vi "RT Main.vi"() -> ()   [LabVIEW 2021]
doc: "Demonstrates the use of Transmission Control Protocol (TCP) to continuously receive LED status from the host computer."
uses:
  <vilib>/myRIO/Express VI/Onboard Devices/LED/LED Express VI.xnode
  <vilib>/myRIO/Instrument Drivers/Onboard IO/DIO/vis/Write.vi
  <vilib>/myRIO/Instrument Drivers/Onboard IO/DIO/DIO.lvlib
  <vilib>/myRIO/Common/Instrument Driver Framework/myRIO v1.0/DIO/typedefs/DIO Channels Enum.ctl
  <vilib>/myRIO/Common/Instrument Driver Framework/myRIO v1.0/DIO/typedefs/DIO Channels List.ctl
  <vilib>/myRIO/Common/Instrument Driver Framework/Utilities/typedefs/Generic FPGA Reference.ctl
  <vilib>/myRIO/Common/Instrument Driver Framework/Utilities/typedefs/myRIO v1.0 Reference.ctl
  <vilib>/myRIO/Common/Instrument Driver Framework/Utilities/typedefs/Hardware Version Enum.ctl
  <vilib>/myRIO/Common/Instrument Driver Framework/Utilities/typedefs/myRIO Generic Hardware Reference.ctl
  <vilib>/myRIO/Instrument Drivers/Onboard IO/DIO/typedefs/DIO Reference.ctl
  <vilib>/myRIO/Instrument Drivers/Onboard IO/DIO/vis/myRIO DIO Open.xnode
  <vilib>/myRIO/Common/Instrument Driver Framework/Utilities/vis/Is FPGA Ref Available.vi
  <vilib>/myRIO/Instrument Drivers/Utilities/Utilities.lvlib
  <vilib>/myRIO/Common/Instrument Driver Framework/myRIO v1.0/DIO/vis/myRIO v1.2 Open DIO.vi
  <vilib>/userdefined/High Color/nirio_resource_hc.ctl
panel:
  out "LED Status":bool[](array[boolean])
  out "error out":errorcluster
  in  "Host IP Address":string="172.22.11.1"
  in  "Stop":bool
  # "Overview: Demonstrates the use of Transmission Control Protocol (TCP) to continuously receive LED status from the host computer.\nInstructions:\n1. Ensure Desktop Main.vi is already running.\n2. Verify the value of Host IP Address. If it is incorrect, specify the correct value.\n3. Observe the LEDs on the myRIO device and the value of LED Status on this VI. They change when the value of Tank on Desktop Main.vi changes.\n4. Click Stop to stop this VI. Stopping this VI also terminates the running of Desktop Main.vi."
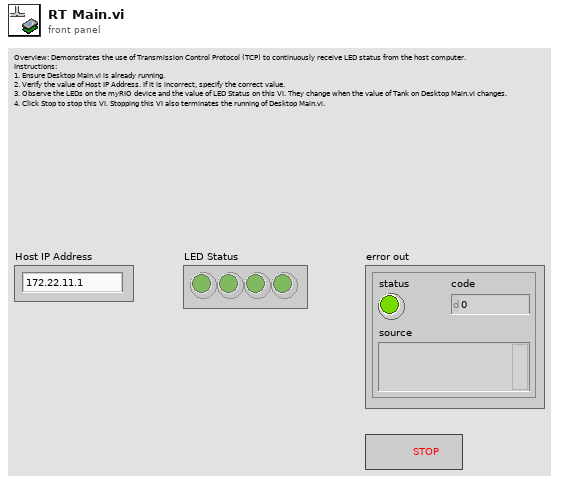
[diagram p1: front panel]
types:
  T1 = typedef "DIO.lvlib/DIO Reference.ctl" = cluster{"myRIO Reference":T2, "DIO Channels List":T6}
  T2 = typedef "myRIO Generic Hardware Reference.ctl" = cluster{"myRIO Model":T3, "myRIO Hardware Reference":T4}
  T3 = typedef "Hardware Version Enum.ctl" = enum16{"Unknown", "myRIO-1900", "myRIO-1950", "roboRIO", "NI ELVIS RIO CM", "ELVIS III"}
  T4 = typedef "myRIO v1.0 Reference.ctl" = cluster{"Generic FPGA Reference":T5, "Allow multiple opens":bool}
  T5 = typedef "Generic FPGA Reference.ctl" = refnum<k20>
  T6 = typedef "DIO Channels List.ctl" = T7[]
  T7 = typedef "DIO Channels Enum.ctl" = enum16{"Not Connected", "C/DIO0", "C/DIO1", "C/DIO2", "C/DIO3", "C/DIO4", "C/DIO5", "C/DIO6", "C/DIO7", "A/DIO0", "A/DIO1", "A/DIO2", "A/DIO3", "A/DIO4", "A/DIO5", "A/DIO6", "A/DIO7", "A/DIO8", "A/DIO9", "A/DIO10", "A/DIO11", "A/DIO12", "A/DIO13", "A/DIO14", "A/DIO15", "A/DIO16", "A/DIO17", "A/DIO18", "A/DIO19", "B/DIO0", "B/DIO1", "B/DIO2", "B/DIO3", "B/DIO4", "B/DIO5", "B/DIO6", "B/DIO7", "B/DIO8", "B/DIO9", "B/DIO10", "B/DIO11", "B/DIO12", "B/DIO13", "B/DIO14", "B/DIO15", "B/DIO16", "B/DIO17", "B/DIO18", "B/DIO19", "LED0", "LED1", "LED2", "LED3", "Button0", "DIO/DIO0", "DIO/DIO1", "DIO/DIO2", "DIO/DIO3", "DIO/DIO4", "DIO/DIO5", "DIO/DIO6", "DIO/DIO7", "DIO/DIO8", "DIO/DIO9", "SPI/CS0", "SPI/CS1", "SPI/CS2", "SPI/CS3", "LED RADIO (Green)", "LED RADIO (Red)", "LED COMM (Green)", "LED COMM (Red)", "LED MODE (Green)", "LED MODE (Red)"}
  T8 = typedef "nirio_resource_hc.ctl" = tag
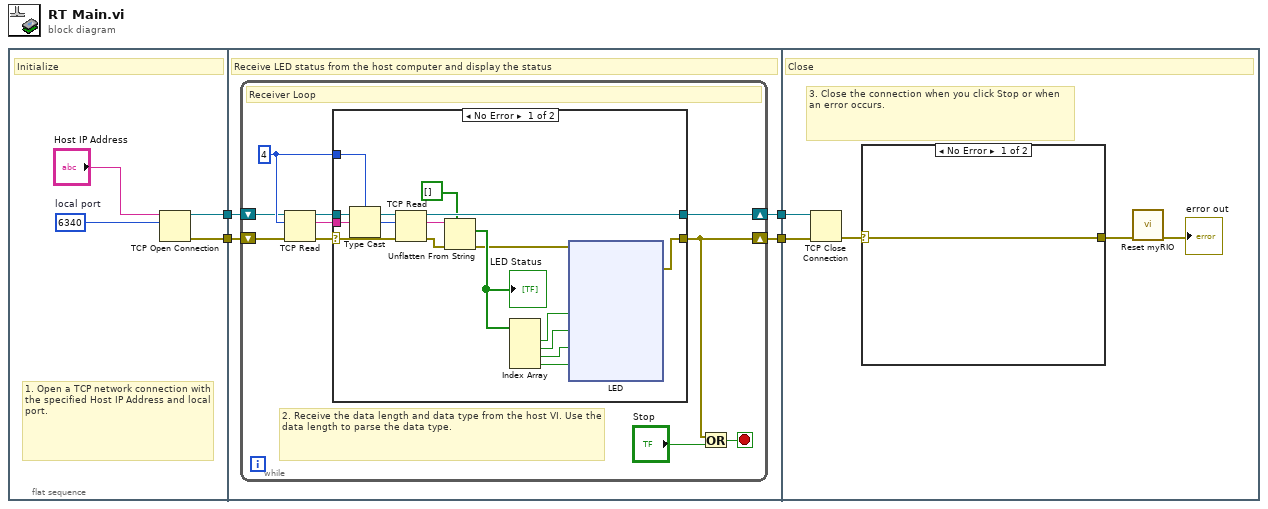
[diagram p0: block diagram]
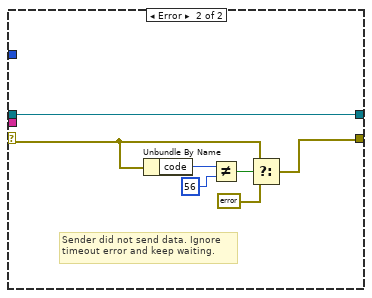
[diagram p2: hidden frame]
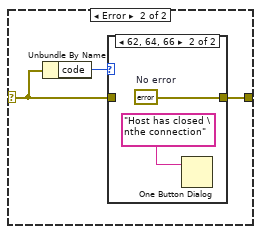
[diagram p3: hidden frame]
diagram:
  n1 = flat-sequence {
    tunnel: [w6] -> w2
    tunnel: [w5] -> w1
    tunnel: [w12] -> w4
    tunnel: [w11] -> w3
    tunnel: w2 -> [w10]
    tunnel: w1 -> [w9]
    tunnel: w4 -> [w88]
    tunnel: w3 -> [w87]
    frame #0 {
      w7 = u16 6340  # local port
      # "1. Open a TCP network connection with the specified Host IP Address and local port."
      # "Initialize"
      n2 = TCP Open Connection(address="Host IP Address", remote port or service name=w7) -> (connection ID=w6:refnum<k5>, error out=w5:errorcluster)  [unwired: 3 in]
    }
    frame #1 {
      # "Receive LED status from the host computer and display the status"
      n3 = while {
        shift-right: [w15] -> w12
        shift-left: w10 -> [w17]
        shift-right: [w14] -> w11
        shift-left: w9 -> [w16]
        stop <- w21 stop-if-true
        w19 = 4 ("bytes to read")
        # "2. Receive the data length and data type from the host VI. Use the data length to parse the data type."
        # "Receiver Loop"
        n4 = TCP Read(connection ID=w17, bytes to read=w19, error in (no error)=w16) -> (connection ID out=w18:refnum<k5>, data out=w20:string, error out=w13:errorcluster)  [unwired: 2 in]
        n5 = case shown="No Error" w13 {
          selector: w13 -> [w25 w79]
          tunnel: w20 -> [w38 _]
          tunnel: w19 -> [w37 _]
          tunnel: w18 -> [w35 w77]
          tunnel: [w32 w77] -> w15
          tunnel: [w23 w78] -> w14
          frame No Error {
            n6 = Type Cast(type=w37, x=w38) -> (*(type *) &x=w36:i32)
            n7 = TCP Read(connection ID=w35, bytes to read=w36, error in (no error)=w25) -> (connection ID out=w32:refnum<k5>, data out=w34:string, error out=w33:errorcluster)  [unwired: 2 in]
            n8 = Unflatten From String(type=bool[] [], binary string=w34, error in (no error)=w33) -> (value=w30:bool[], error out=w24:errorcluster)  [unwired: 2 in, 1 out]
            "LED Status" <- w30
            n9 = Index Array(array=w30) -> (element #1=w29:bool, element #2=w28:bool, element #3=w27:bool, element #4=w26:bool)  [unwired: 4 in]
            n10 = xnode "LED"("LED0"=w29, "LED1"=w28, "LED2"=w27, "LED3"=w26, "error in (no error)"=w24) -> ("error out"=w23:errorcluster)
          }
          frame Error {
            # "Sender did not send data. Ignore \ntimeout error and keep waiting."
            n11 = Unbundle By Name(w79) -> ("code"=w82:i32)
            n12 = Not Equal?(x=w82, y=56) -> (x != y?=w83:bool)
            n13 = Select(t=w79, s=w83, f=errorcluster {"status"=FALSE, "code"=0, "source"=""} ("error out")) -> (s? t:f=w78:errorcluster)
          }
        }
        n14 = Or(x=w14, y="Stop") -> (x .or. y?=w21:bool)
      }
    }
    frame #2 {
      # "3. Close the connection when you click Stop or when an error occurs."
      # "Close"
      n15 = TCP Close Connection(connection ID=w88, error in (no error)=w87) -> (error out=w85:errorcluster)  [unwired: 1 in, 1 out]
      n16 = case shown="No Error" w85 {
        selector: w85 -> [w89 w90]
        tunnel: [w89 w91] -> w84
        frame No Error {
        }
        frame Error {
          n17 = Unbundle By Name(w90) -> ("code"=w92:i32)
          n18 = case shown="62, 64, 66" w92 {
            tunnel: w90 -> [w93 _]
            tunnel: [w93 w94] -> w91
            frame Default {
            }
            frame 62, 64, 66 {
              w94 = errorcluster {"status"=FALSE, "code"=0, "source"=""}  # No error
              n19 = One Button Dialog(message="Host has closed \nthe connection") -> ()  [unwired: 1 in, 1 out]
            }
          }
        }
      }
      n20 = call <vilib>:"Reset myRIO.vi"("error in (no error)"=w84) -> ("error out"=→"error out":errorcluster)  [unwired: 10 in]
    }
  }
